vi "Set TDMS WFM Properties.vi"(1 "Settings":string[](array[string]), 4 "Configuration":variant, 5 "dt":dbl, 6 "Scaling coefficients":dbl[][](array[numeric]), 7 "t0":dbl, 8 "error in (no error)":errorcluster, 9 "Channel names":string[](array[string]), 10 "Group name":string="p", 11 "tdms file":refnum<k34>) -> (0 "error out":errorcluster, 3 "tdms file out":refnum<k34>)   [LabVIEW 2019]
uses:
  <vilib>/Utility/tdmsutil.llb/TDMS Create Scaling Information (Linear).vi
  8a8c82c9-4748-4a37-8d6f-9f2ec094c772.vi
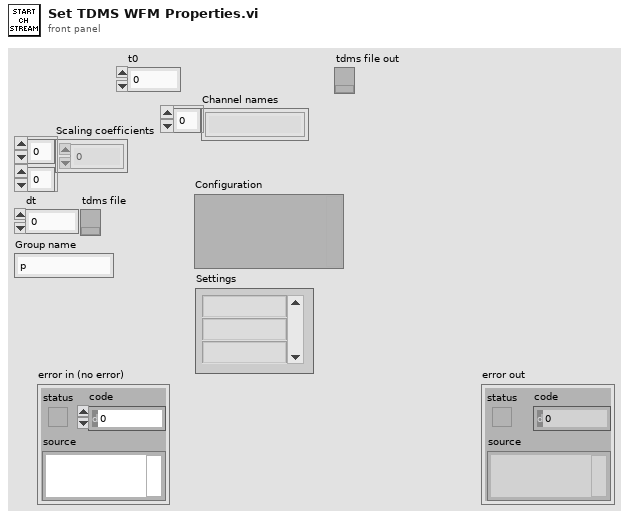
[diagram p1: front panel]
types:
  T1 = cluster{"slope":dbl, "y intercept":dbl, "input source":i32}
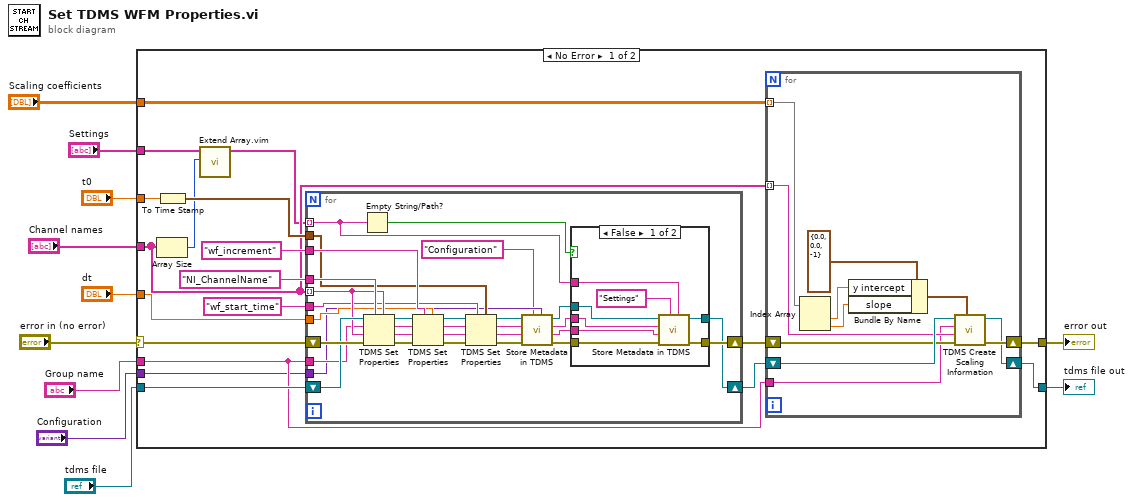
[diagram p0: block diagram]
diagram:
  n1 = case shown="No Error" "error in (no error)" {
    selector: "error in (no error)" -> [w30 w84]
    tunnel: [w18 w84] -> w10
    tunnel: "tdms file" -> [w25 w83]
    tunnel: "dt" -> [w24 _]
    tunnel: "t0" -> [w23 _]
    tunnel: "Scaling coefficients" -> [w17 _]
    tunnel: "Group name" -> [w22 _]
    tunnel: "Channel names" -> [w15 _]
    tunnel: [w19 w83] -> w3
    tunnel: "Configuration" -> [w16 _]
    tunnel: "Settings" -> [w12 _]
    frame No Error {
      n2 = Array Size(array=w15) -> (size(s)=w14:i32)
      n3 = To Time Stamp(1:w23) -> (0:w27:timestamp)
      n4 = call "Extend Array.vim"("Extend to size"=w14, "Array in"=w12) -> ("Array out"=w13:string[])  [unwired: 8 in, 1 out]
      n5 = for {
        tunnel: "NI_ChannelName" -> [w69]
        tunnel: w15 -> [w68] mode=indexing
        tunnel: w24 -> [w67]
        tunnel: w27 -> [w66]
        tunnel: "wf_start_time" -> [w65]
        shift-right: [w47] -> w21
        shift-left: w30 -> [w72]
        shift-right: [w46] -> w20
        shift-left: w25 -> [w71]
        tunnel: "wf_increment" -> [w70]
        tunnel: w22 -> [w56]
        tunnel: w16 -> [w52]
        tunnel: w13 -> [w43] mode=indexing
        n6 = Empty String/Path?(string/path=w43) -> (empty?=w42:bool)
        n7 = TDMS Set Properties(5:w68, 7:w69, 8:w72, 9:w68, 10:w56, 11:w71) -> (0:w64:errorcluster, 1:w61:string, 2:w63:string, 3:w62:refnum<k34>)
        n8 = TDMS Set Properties(5:w67, 7:w70, 8:w64, 9:w61, 10:w63, 11:w62) -> (0:w60:errorcluster, 1:w59:string, 2:w58:string, 3:w57:refnum<k34>)
        n9 = TDMS Set Properties(5:w66, 7:w65, 8:w60, 9:w59, 10:w58, 11:w57) -> (0:w51:errorcluster, 1:w53:string, 2:w54:string, 3:w55:refnum<k34>)
        n10 = call "Store Metadata in TDMS.vi"("Value"=w52, "name"="Configuration" ("property names"), "Error In"=w51, "channel name"=w53, "group name"=w54, "tdms file"=w55) -> ("Error Out"=w48:errorcluster, "channel name out"=w44:string, "group name out"=w45:string, "tdms file out"=w49:refnum<k34>)  [unwired: 2 in]
        n11 = case shown="False" w42 {
          tunnel: w49 -> [w80 w82]
          tunnel: w48 -> [w79 w81]
          tunnel: [w78 w81] -> w47
          tunnel: [w77 w82] -> w46
          tunnel: w43 -> [w75 _]
          tunnel: w45 -> [w74 _]
          tunnel: w44 -> [w73 _]
          frame False {
            n12 = call "Store Metadata in TDMS.vi"("Value"=w75, "name"="Settings" ("property names"), "Error In"=w79, "channel name"=w73, "group name"=w74, "tdms file"=w80) -> ("Error Out"=w78:errorcluster, "tdms file out"=w77:refnum<k34>)  [unwired: 2 in, 2 out]
          }
          frame True {
          }
        }
      }
      n13 = for {
        tunnel: w17 -> [w39] mode=indexing
        tunnel: w15 -> [w33] mode=indexing
        shift-right: [w37] -> w18
        shift-left: w21 -> [w32]
        shift-right: [w36] -> w19
        shift-left: w20 -> [w34]
        tunnel: w22 -> [w31]
        n14 = Index Array(array=w39) -> (element #1=w41:dbl, element #2=w35:dbl)  [unwired: 2 in]
        n15 = Bundle By Name(cluster=T1 {"slope"=0.0, "y intercept"=0.0, "input source"=-1} ("linear scale"), "y intercept"=w41, "slope"=w35) -> (w40:T1)
        n16 = call-poly <vilib>:"TDMS Create Scaling Information.vi"("linear scale"=w40, "error in (no error)"=w32, "channel name"=w33, "group name"=w31, "tdms file"=w34) -> ("error out"=w37:errorcluster, "tdms file out"=w36:refnum<k34>)  [unwired: 2 in, 3 out]
      }
    }
    frame Error {
    }
  }
  "error out" <- w10
  "tdms file out" <- w3
